vi "TwoBendingRootSubVi.vi"(0 "x node":i32, 1 "y node":i32, 2 "t":dbl, 3 "u":dbl, 4 "amp 1":dbl, 5 "amp 2":dbl, 6 "x":dbl, 7 "nL":dbl, 9 "phi 1":dbl, 11 "phi 2":dbl) -> (14 "BendRoot":dbl, 19 "Bend":dbl)   [LabVIEW 2017]
panel:
  out "x/y":dbl
  # "Salmon Parameters (amp1 = 0.0488,amp2 = 0.0832,phi=0.8499,c=0.0281,u=62.8319)"
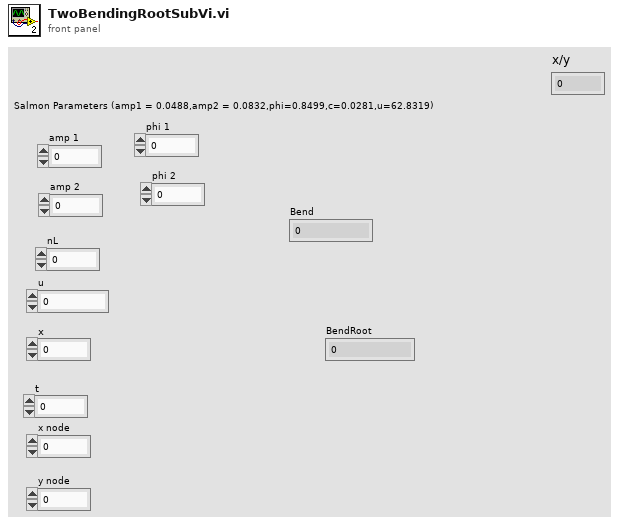
[diagram p1: front panel]
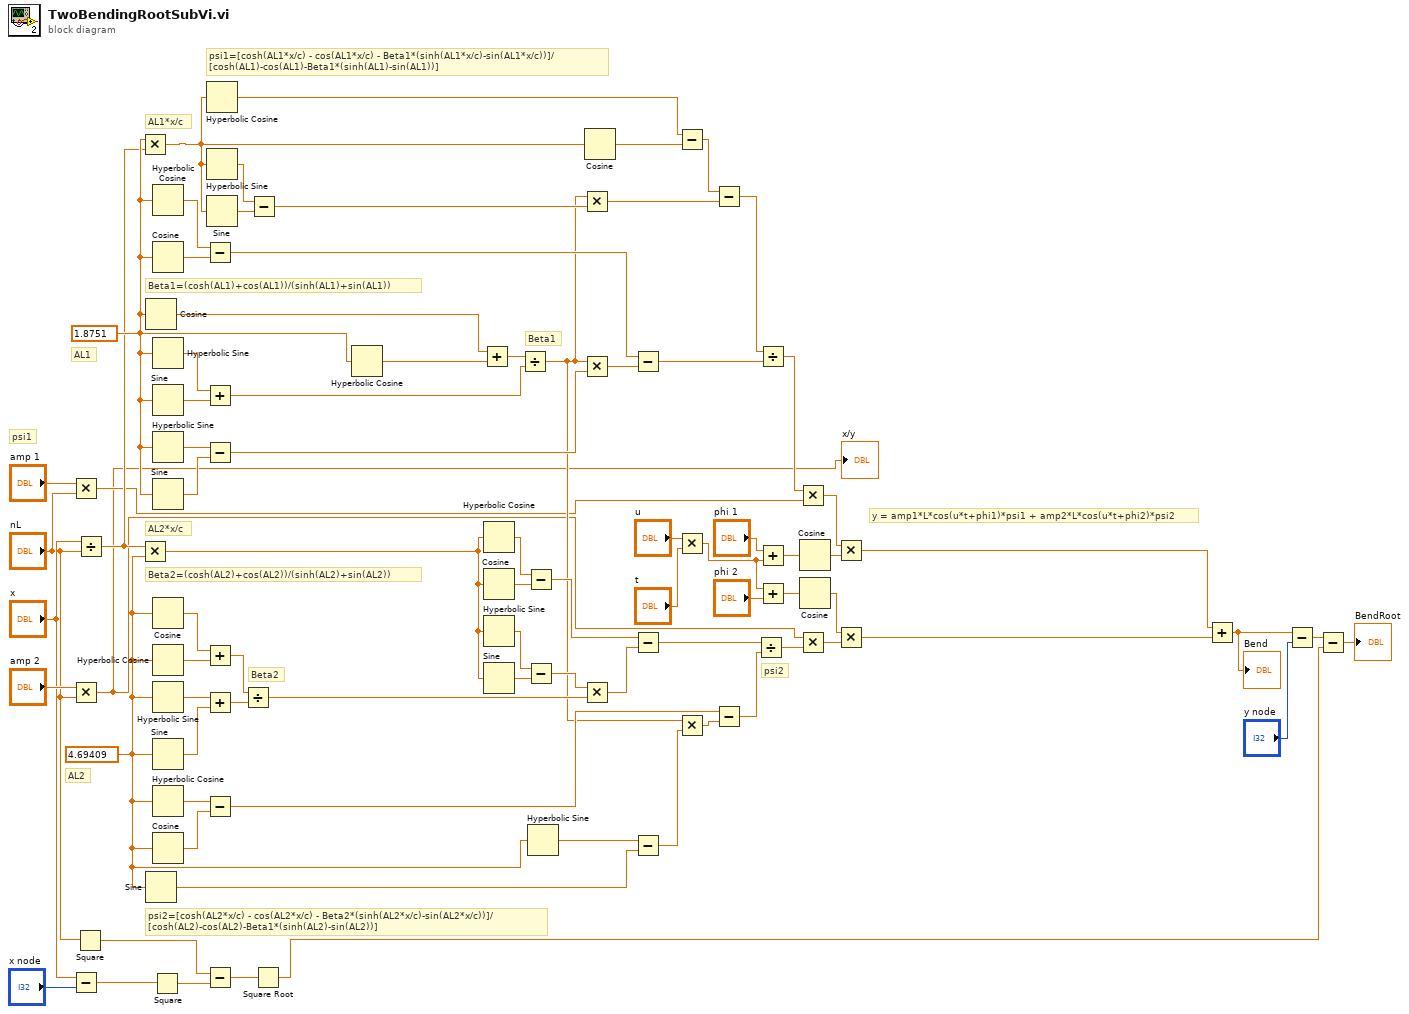
[diagram p0: block diagram]
diagram:
  w41 = 4.69409
  w63 = 1.8751
  # "psi2"
  # "psi1"
  # "AL2*x/c"
  # "AL1*x/c"
  # "psi2=[cosh(AL2*x/c) - cos(AL2*x/c) - Beta2*(sinh(AL2*x/c)-sin(AL2*x/c))]/\n[cosh(AL2)-cos(AL2)-Beta1*(sinh(AL2)-sin(AL2))]"
  # "psi1=[cosh(AL1*x/c) - cos(AL1*x/c) - Beta1*(sinh(AL1*x/c)-sin(AL1*x/c))]/\n[cosh(AL1)-cos(AL1)-Beta1*(sinh(AL1)-sin(AL1))]"
  # "y = amp1*L*cos(u*t+phi1)*psi1 + amp2*L*cos(u*t+phi2)*psi2"
  # "Beta2=(cosh(AL2)+cos(AL2))/(sinh(AL2)+sin(AL2))"
  # "Beta1=(cosh(AL1)+cos(AL1))/(sinh(AL1)+sin(AL1))"
  # "Beta2"
  # "Beta1"
  # "AL2"
  # "AL1"
  n1 = Multiply(x="amp 1", y="nL") -> (x*y=w2:dbl)
  n2 = Multiply(x="amp 2", y="nL") -> (x*y=w1:dbl)
  "x/y" <- w1
  n3 = Subtract(x="x", y="x node") -> (x-y=w18:dbl)
  n4 = Square(x="nL") -> (x^2=w15:dbl)
  n5 = Divide(x="x", y="nL") -> (x/y=w6:dbl)
  n6 = Multiply(x=w63, y=w6) -> (x*y=w7:dbl)
  n7 = Multiply(x=w6, y=w41) -> (x*y=w42:dbl)
  n8 = Cosine(x=w63) -> (cos(x)=w81:dbl)
  n9 = Sine(x=w41) -> (sin(x)=w43:dbl)
  n10 = Square(x=w18) -> (x^2=w14:dbl)
  n11 = Hyperbolic Cosine(1:w63) -> (0:w62:dbl)
  n12 = Cosine(x=w63) -> (cos(x)=w61:dbl)
  n13 = Hyperbolic Sine(1:w63) -> (0:w80:dbl)
  n14 = Sine(x=w63) -> (sin(x)=w79:dbl)
  n15 = Hyperbolic Sine(1:w63) -> (0:w60:dbl)
  n16 = Sine(x=w63) -> (sin(x)=w59:dbl)
  n17 = Cosine(x=w41) -> (cos(x)=w77:dbl)
  n18 = Hyperbolic Cosine(1:w41) -> (0:w78:dbl)
  n19 = Hyperbolic Sine(1:w41) -> (0:w76:dbl)
  n20 = Sine(x=w41) -> (sin(x)=w75:dbl)
  n21 = Hyperbolic Cosine(1:w41) -> (0:w46:dbl)
  n22 = Cosine(x=w41) -> (cos(x)=w45:dbl)
  n23 = Subtract(x=w62, y=w61) -> (x-y=w56:dbl)
  n24 = Add(x=w80, y=w79) -> (x+y=w73:dbl)
  n25 = Subtract(x=w60, y=w59) -> (x-y=w58:dbl)
  n26 = Add(x=w77, y=w78) -> (x+y=w72:dbl)
  n27 = Add(x=w76, y=w75) -> (x+y=w71:dbl)
  n28 = Subtract(x=w46, y=w45) -> (x-y=w25:dbl)
  n29 = Subtract(x=w15, y=w14) -> (x-y=w16:dbl)
  n30 = Hyperbolic Cosine(1:w7) -> (0:w67:dbl)
  n31 = Hyperbolic Sine(1:w7) -> (0:w70:dbl)
  n32 = Sine(x=w7) -> (sin(x)=w69:dbl)
  n33 = Divide(x=w72, y=w71) -> (x/y=w36:dbl)
  n34 = Subtract(x=w70, y=w69) -> (x-y=w68:dbl)
  n35 = Square Root(x=w16) -> (sqrt(x)=w13:dbl)
  n36 = Hyperbolic Cosine(1:w63) -> (0:w82:dbl)
  n37 = Add(x=w81, y=w82) -> (x+y=w74:dbl)
  n38 = Hyperbolic Cosine(1:w42) -> (0:w48:dbl)
  n39 = Cosine(x=w42) -> (cos(x)=w47:dbl)
  n40 = Hyperbolic Sine(1:w42) -> (0:w50:dbl)
  n41 = Sine(x=w42) -> (sin(x)=w49:dbl)
  n42 = Divide(x=w74, y=w73) -> (x/y=w22:dbl)
  n43 = Subtract(x=w48, y=w47) -> (x-y=w28:dbl)
  n44 = Subtract(x=w50, y=w49) -> (x-y=w35:dbl)
  n45 = Hyperbolic Sine(1:w41) -> (0:w44:dbl)
  n46 = Multiply(x=w22, y=w68) -> (x*y=w64:dbl)
  n47 = Multiply(x=w22, y=w58) -> (x*y=w57:dbl)
  n48 = Multiply(x=w35, y=w36) -> (x*y=w27:dbl)
  n49 = Cosine(x=w7) -> (cos(x)=w66:dbl)
  n50 = Subtract(x=w56, y=w57) -> (x-y=w8:dbl)
  n51 = Subtract(x=w28, y=w27) -> (x-y=w26:dbl)
  n52 = Subtract(x=w44, y=w43) -> (x-y=w24:dbl)
  n53 = Subtract(x=w67, y=w66) -> (x-y=w65:dbl)
  n54 = Multiply(x="u", y="t") -> (x*y=w40:dbl)
  n55 = Multiply(x=w22, y=w24) -> (x*y=w23:dbl)
  n56 = Subtract(x=w65, y=w64) -> (x-y=w9:dbl)
  n57 = Subtract(x=w25, y=w23) -> (x-y=w29:dbl)
  n58 = Divide(x=w26, y=w29) -> (x/y=w30:dbl)
  n59 = Divide(x=w9, y=w8) -> (x/y=w5:dbl)
  n60 = Add(x="phi 1", y=w40) -> (x+y=w4:dbl)
  n61 = Add(x=w40, y="phi 2") -> (x+y=w37:dbl)
  n62 = Multiply(x=w5, y=w2) -> (x*y=w51:dbl)
  n63 = Multiply(x=w1, y=w30) -> (x*y=w31:dbl)
  n64 = Cosine(x=w4) -> (cos(x)=w3:dbl)
  n65 = Cosine(x=w37) -> (cos(x)=w32:dbl)
  n66 = Multiply(x=w51, y=w3) -> (x*y=w34:dbl)
  n67 = Multiply(x=w32, y=w31) -> (x*y=w33:dbl)
  n68 = Add(x=w34, y=w33) -> (x+y=w10:dbl)
  "Bend" <- w10
  n69 = Subtract(x=w10, y="y node") -> (x-y=w19:dbl)
  n70 = Subtract(x=w19, y=w13) -> (x-y=→"BendRoot":dbl)
